vi "Read Macro.vi"(8 "error in (no error)":errorcluster, 11 "File Path":path) -> (0 "error out":errorcluster, 3 "Macro":T1)   [LabVIEW 2023]
doc: "Loads the macro defined by <B>Macro Name</B> from an INI file located in <B>App Data Directory</B>."
uses:
  CTLs/Macro Cluster V3.ctl
  CTLs/Macro Config V3.ctl
  CTLs/Step V3.ctl
  CTLs/Step Type V3.ctl
  <vilib>/Utility/error.llb/Error Cluster From Error Code.vi
  <vilib>/ErrorRing/Error Ring.xnode
  <vilib>/Utility/config.llb/NI_LVConfig.lvlib
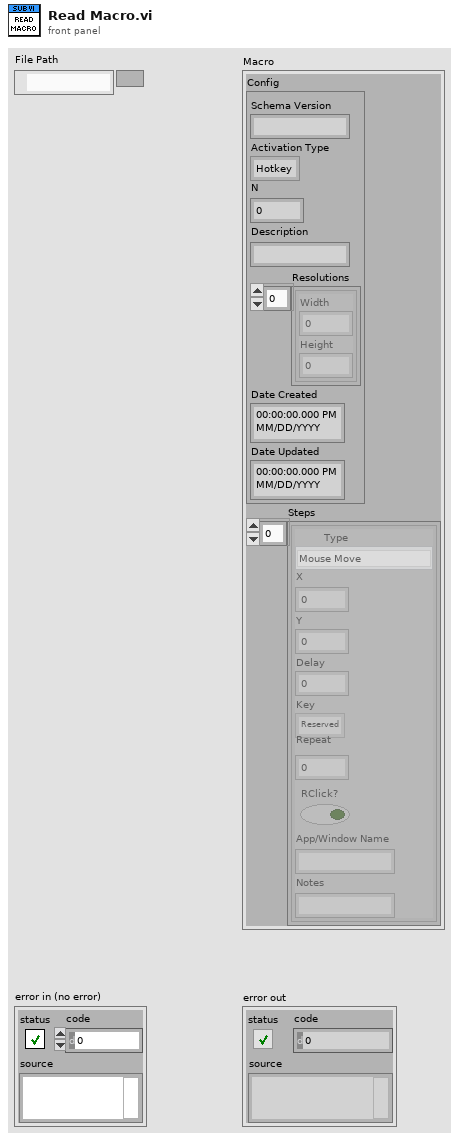
[diagram p1: front panel]
types:
  T1 = typedef "Macro Cluster V3.ctl" = cluster{"Config":T2, "Steps":T3[]}
  T2 = typedef "Macro Config V3.ctl" = cluster{"Schema Version":string, "Activation Type":enum32{"Hotkey", "Automatic"}, "N":i32, "Description":string, "Resolutions":cluster{"Width":i16, "Height":i16}[], "Date Created":timestamp, "Date Updated":timestamp}
  T3 = typedef "Step V3.ctl" = cluster{"Type":T4, "X":i32, "Y":i32, "Delay":i32, "Key":u8, "Repeat":i32, "RClick?":bool, "App/Window Name":string, "Notes":string}
  T4 = typedef "Step Type V3.ctl" = enum16{"Mouse Move", "Mouse Click", "Key Press", "Wait", "Mouse Down", "Mouse Up", "Key Down", "Key Up", "Run Application", "Maximize Window", "Restore Window", "Minimize Window", "Close Window", "Bring Window to Front", "Send Window to Back"}
  T5 = typedef "NI_LVConfig.lvlib/Config Data RefNum.ctl" = refnum<k1>
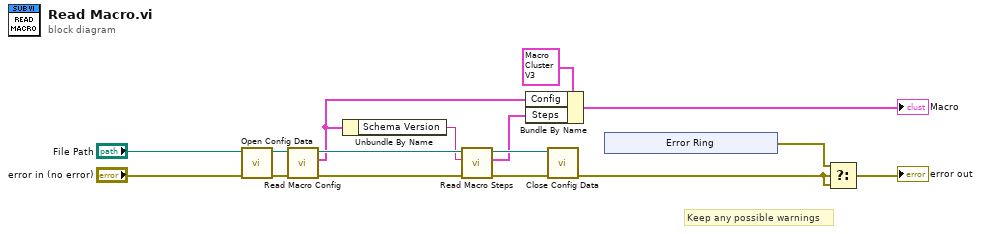
[diagram p0: block diagram]
diagram:
  # "Keep any possible warnings"
  n1 = call <vilib>:"Open Config Data.vi"("error in (no error)"="error in (no error)", "configuration file path"="File Path") -> ("error out"=w12:errorcluster, "refnum"=w13:T5)  [unwired: 7 in, 1 out]
  n2 = call "Read Macro Config.vi"("error in (no error)"=w12, "refnum"=w13) -> ("error out"=w10:errorcluster, "Macro Config"=w3:T2, "refnum out"=w11:T5)  [unwired: 7 in]
  n3 = Unbundle By Name(w3) -> ("Schema Version"=w2:string)
  n4 = call "Read Macro Steps.vi"("error in (no error)"=w10, "Schema Version"=w2, "refnum"=w11) -> ("error out"=w9:errorcluster, "Macro Steps"=w6:T3[], "refnum out"=w7:T5)  [unwired: 6 in]
  n5 = Bundle By Name(cluster=T1 {"Config"={"Schema Version"="", "Activation Type"=enum."Hotkey", "N"=0, "Description"="", "Resolutions"=[], "Date Created"=timestamp(0 s since 1904-01-01), "Date Updated"=timestamp(0 s since 1904-01-01)}, "Steps"=[]} ("Macro"), "Config"=w3, "Steps"=w6) -> (→"Macro":T1)
  n6 = call <vilib>:"Close Config Data.vi"("error in (no error)"=w9, "refnum"=w7) -> ("error out"=w8:errorcluster)  [unwired: 8 in, 1 out]
  n7 = xnode "Error Ring"() -> ("error out"=w15:errorcluster)
  n8 = Select(t=w15, s=w8, f=w8) -> (s? t:f=→"error out":errorcluster)
